vi "LVUSBRH2_VISA_SUB_parseResponseString_Getrh.vi"(11 "recv string":string=":23.81, 43.20, C8\n") -> (2 "data[]":dbl[](array[numeric]), 4 "data string[]":string[](array[string]))   [LabVIEW 2020]
panel:
  # "温度 ℃\n相対湿度 RH%"
  # "USBRH2の温度・湿度取得コマンド getrh[cr|lf] の応答文字列を解析する\n\nUSBRH2についてはこちら\nhttps://strawberry-linux.com/catalog/items?code=52031"
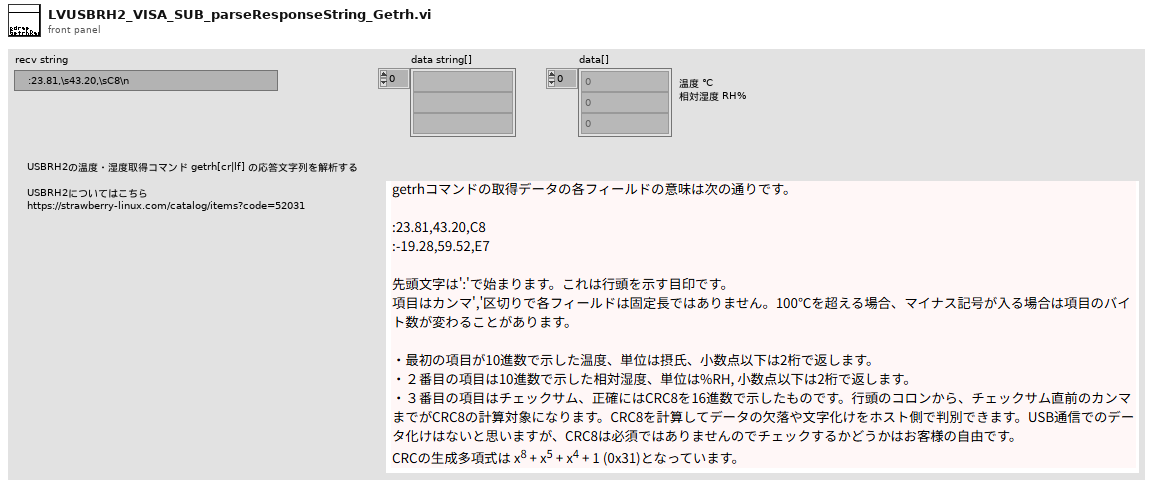
[diagram p1: front panel]
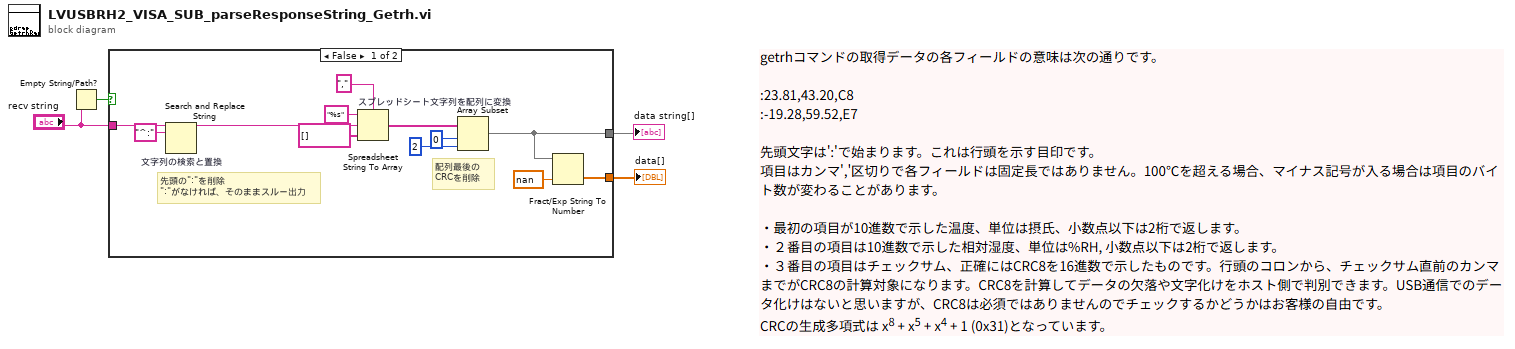
[diagram p0: block diagram]
diagram:
  n1 = Empty String/Path?(string/path="recv string") -> (empty?=w1:bool)
  n2 = case shown="FALSE" w1 {
    tunnel: "recv string" -> [w14 _]
    tunnel: [w8 _] -> w4
    tunnel: [w6 _] -> w3
    frame False {
      # "配列最後の\nCRCを削除"
      # "先頭の\":\"を削除\n\":\"がなければ、そのままスルー出力"
      n3 = Search and Replace String "文字列の検索と置換"(input string=w14, search string="^:" ("検索文字列")) -> (result string=w12:string)  [unwired: 6 in, 3 out]
      n4 = Spreadsheet String To Array "スプレッドシート文字列を配列に変換"(delimiter (Tab)=",", format string="%s" ("形式文字列"), spreadsheet string=w12, array type (2D Dbl)=string[] [] ("配列タイプ (2次元Dbl)")) -> (array=w11:string[])
      n5 = Array Subset(array=w11, index=0 ("長さ"), length=2 ("長さ")) -> (w8:string[])
      n6 = Fract/Exp String To Number(string=w8, default (0 dbl)=nan ("デフォルト (0 DBL)")) -> (number=w6:dbl[])  [unwired: 2 in, 1 out]
    }
    frame True {
    }
  }
  "data string[]" <- w4
  "data[]" <- w3
